vi "buil_temp_array.vi"() -> ()   [LabVIEW 2018]
uses:
  <vilib>/Platform/TimedLoop/XDataNode/timing_clust.ctl
  <vilib>/Platform/TimedLoop/XDataNode/nitl_modes.ctl
  <vilib>/Platform/TimedLoop/XDataNode/wakeup.ctl
  <vilib>/rvi/Emulation/niFpgaSctlEmulationGetInTimedLoop.vi
  <vilib>/rvi/Emulation/niFpgaEmulationReportErrorSimple.vi
  <vilib>/rvi/Emulation/niFpgaGetClockAttributes.vi
  <vilib>/rvi/Emulation/niFpgaCriticalErrorInLSC.vi
  <vilib>/Platform/TimedLoop/XDataNode/XDataNode.xnode
  <vilib>/Platform/TimedLoop/XDataNode/XDNodeRunTimeDep.lvlib
panel:
  out "Array 2":fxp<+/-,35,16>[](array[numeric])
  in  "Array":fxp<+/-,24,5>[](array[numeric])=[0.0, 0.0, 0.0, 0.0, 0.0, 0.0, 0.0, 0.0, 0.0, 0.0, 0.0, 0.0, 0.0, 0.0, 0.0]
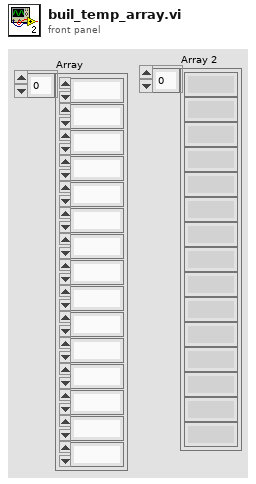
[diagram p1: front panel]
types:
  T1 = typedef "XDNodeRunTimeDep.lvlib/timing_clust.ctl" = cluster{"Expected End [f-1]":u64, "Actual End [f-1]":u64, "Finished Late? [f-1]":bool, "Expected End [i-1]":u64, "Actual End [i-1]":u64, "Finished Late? [i-1]":bool, "Expected Start [i]":u64, "Actual Start [i]":u64, "Expected Start [f]":u64, "Actual Start [f]":u64, "Source Name":string, "Structure Name":string, "Period":i64, "Deadline":i64, "Offset":i64, "Start":i64, "Priority":i32, "Timeout":i32, "Mode":T2, "Wakeup Reason":T3, "Error":errorcluster, "Source Type":string, "Secondary Source Type":string, "Global End Time":u64, "Global Start Time":u64, "Frame Duration":u64, "Iteration Duration":u64, "Assigned CPU":i32, "I/O Scan Engine Mode":u32}
  T2 = typedef "XDNodeRunTimeDep.lvlib/nitl_modes.ctl" = enum32{"No Change", "Process missed periods, maintain original phase", "Discard missed periods, maintain original phase", "Process missed periods, ignore original phase", "Discard missed periods, ignore original phase"}
  T3 = typedef "XDNodeRunTimeDep.lvlib/wakeup.ctl" = enum32{"Normal", "Aborted", "Asynchronous wakeup", "Timing source error", "Timed loop error", "Timeout"}
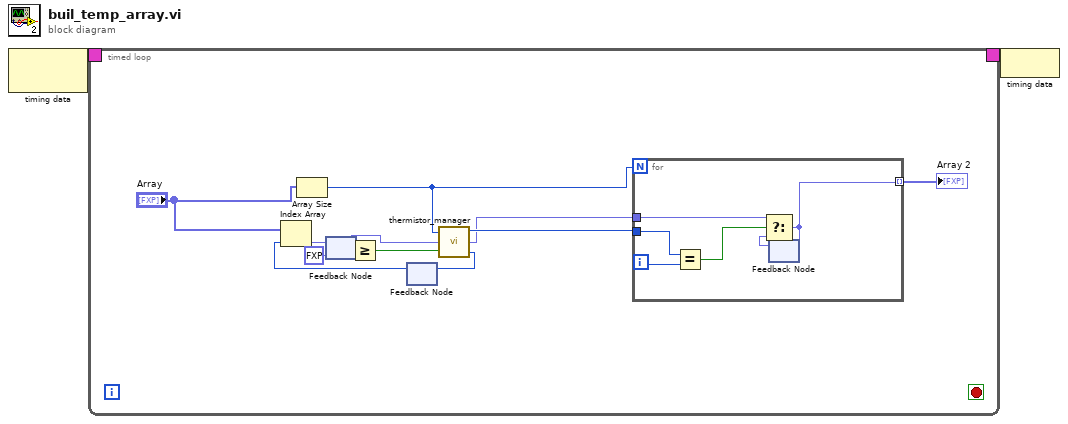
[diagram p0: block diagram]
diagram:
  n1 = node-c288() -> (w2:T1)  [unwired: 1 in]
  n2 = timed-loop {
    timing: w2 -> [_]
    timing-out: [_] -> w1
    stop <- _ stop-if-true
    n3 = Array Size(array="Array") -> (size(s)=w4:i32)
    n4 = feedback #1() -> (w6:fxp<+/-,24,5>)  [unwired: 1 in]
    n5 = Greater Or Equal?(x=w6, y=fxp<+,1,1> 0.0) -> (x >= y?=w8:bool)
    n6 = feedback #2() -> (w12:u16)  [unwired: 1 in]
    n7 = Index Array(array="Array", index=w12) -> (element=w10:fxp<+/-,24,5>)
    n8 = feedback-in #1(w10) -> ()
    n9 = call "thermistor_manager.vi"("input valid"=w8, "V"=w6, "count"=w4) -> ("input_index"=w13:u16, "temperature"=w3:fxp<+/-,32,16>, "output_index"=w7:u16)
    n10 = feedback-in #2(w13) -> ()
    n11 = for {
      N: w4 -> [_]
      tunnel: w7 -> [w19]
      tunnel: [w15] -> w5 mode=indexing
      tunnel: w3 -> [w14]
      i -> [w18]
      n12 = Equal?(x=w19, y=w18) -> (x = y?=w17:bool)
      n13 = feedback #3() -> (w16:fxp<+/-,32,16>)  [unwired: 1 in]
      n14 = Select(t=w14, s=w17, f=w16) -> (s? t:f=w15:fxp<+/-,32,16>)
      n15 = feedback-in #3(w15) -> ()
    }
    "Array 2" <- w5
  }
  n16 = node-c288(w1) -> ()
